vi "Generate Waveforms.vi"(1 "Sound.lvclass":refnum<class "Sound.lvclass">) -> (0 "Waveforms":waveform(dbl)[](array[waveform]))   [LabVIEW 2010, in "Sound.lvclass"]
doc: "This method creates a waveform for the sound to be played.\n\nThis method MUST be overridden by children of Sound."
uses:
  Sound.lvclass
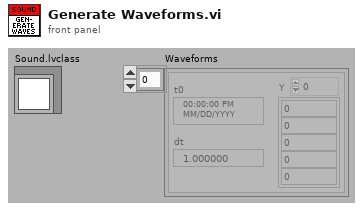
[diagram p1: front panel]
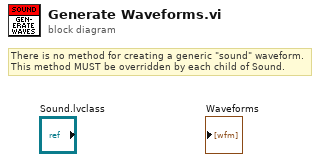
[diagram p0: block diagram]
diagram:
  # "There is no method for creating a generic \"sound\" waveform.  \nThis method MUST be overridden by each child of Sound."
